vi "Read DAQ Parameters.vi"(8 "error in (no error)":errorcluster, 11 "Galvo in":refnum<class "Galvo.lvclass">) -> (0 "error out":errorcluster, 2 "DAQ Parameters":T1={"Points Per A-Scan"=1024, "A-Scans Per B-Scan"=250, "Number of B-Scans"=1, "B-Scans Per Transfer"=1, "Trigger Voltage"=0.0, "Trigger Source"=enum."External", "Trigger Slope"=enum."Rising", "Channel"=enum."Channel 1", "Clock"=enum."Internal Clock", "Bits per Sample"=0.0, "Range"=0.0, "Start Trim"=0, "Stop Trim"=0}, 3 "Galvo out":refnum<class "Galvo.lvclass">)   [LabVIEW 2015, in "Galvo.lvclass"]
uses:
  Galvo.lvclass
  DAQ/DAQ Parameters.ctl
  DAQ/Trigger Source.ctl
  DAQ/Trigger Slope.ctl
  Type Defs/OCT DAQ Channel Data Type.ctl
  DAQ/Clock Control.ctl
  Galvo.lvclass/Galvo.ctl
  DAQ/DAQ Class.lvclass
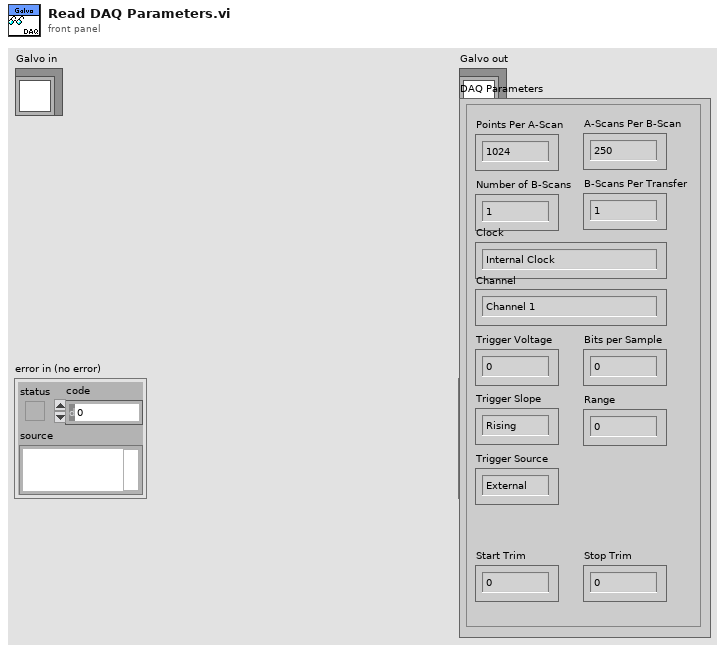
[diagram p1: front panel]
types:
  T1 = typedef "DAQ Class.lvclass/DAQ Parameters.ctl" = cluster{"Points Per A-Scan":u32, "A-Scans Per B-Scan":u32, "Number of B-Scans":u32, "B-Scans Per Transfer":u32, "Trigger Voltage":sgl, "Trigger Source":T2, "Trigger Slope":T3, "Channel":T4, "Clock":T5, "Bits per Sample":dbl, "Range":dbl, "Start Trim":u32, "Stop Trim":u32}
  T2 = typedef "DAQ Class.lvclass/Trigger Source.ctl" = enum16{"External", "Channel A", "Channel B"}
  T3 = typedef "DAQ Class.lvclass/Trigger Slope.ctl" = enum16{"Rising", "Falling"}
  T4 = typedef "OCT DAQ Channel Data Type.ctl" = enum16{"Channel 1", "Channel 2", "Channel 1 and 2"}
  T5 = typedef "DAQ Class.lvclass/Clock Control.ctl" = enum16{"Internal Clock", "External Clock"}
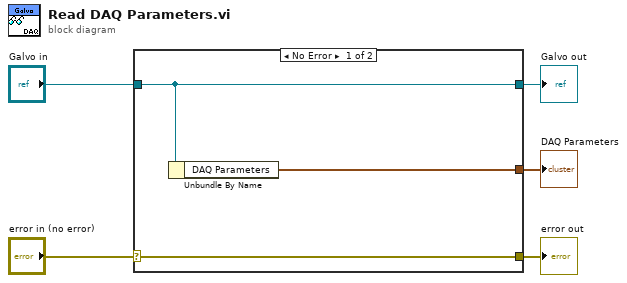
[diagram p0: block diagram]
diagram:
  n1 = case shown="No Error" "error in (no error)" {
    selector: "error in (no error)" -> [w8 w9]
    tunnel: [w8 w9] -> w4
    tunnel: [w7 w10] -> w2
    tunnel: "Galvo in" -> [w7 w10]
    tunnel: [w6 _] -> w1
    frame No Error {
      n2 = Unbundle By Name(w7) -> ("DAQ Parameters"=w6:T1)
    }
    frame Error {
    }
  }
  "error out" <- w4
  "Galvo out" <- w2
  "DAQ Parameters" <- w1
